vi "Create PID VS Name.vi"(10 "PID Number":u16, 11 "PID Name":string) -> (3 "VS Name":string)   [LabVIEW 2015, in "Diagnostics Addon Shared.lvlib"]
uses:
  Diagnostics Addon Shared.lvlib
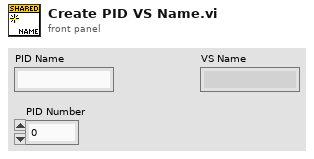
[diagram p1: front panel]
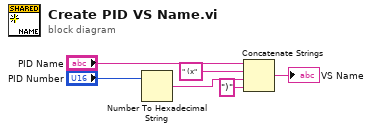
[diagram p0: block diagram]
diagram:
  n1 = Number To Hexadecimal String(2:"PID Number") -> (0:w2:string)  [unwired: 1 in]
  n2 = Concatenate Strings("PID Name", " (x" ("string"), w2, ")" ("string")) -> (→"VS Name":string)
